vi "phase_shift.vi"(8 "reference":refnum<vi>, 9 "Points in Cycle":i32, 10 "Array 2":dbl[](array[numeric]), 11 "Array 1":dbl[](array[numeric])) -> (3 "Phase Shift":dbl)   [LabVIEW 2020]
doc: "Calculates the phase difference of two input arrays\ninput: two one-dimensional arrays, amount of points within one wave, waveform chart reference\noutput: phase difference"
uses:
  <vilib>/Analysis/5stat.llb/RMS (DBL).vi
  <vilib>/Analysis/NI_AALPro.lvlib
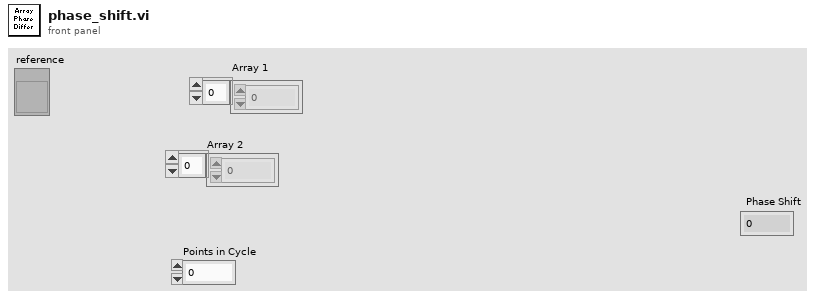
[diagram p1: front panel]
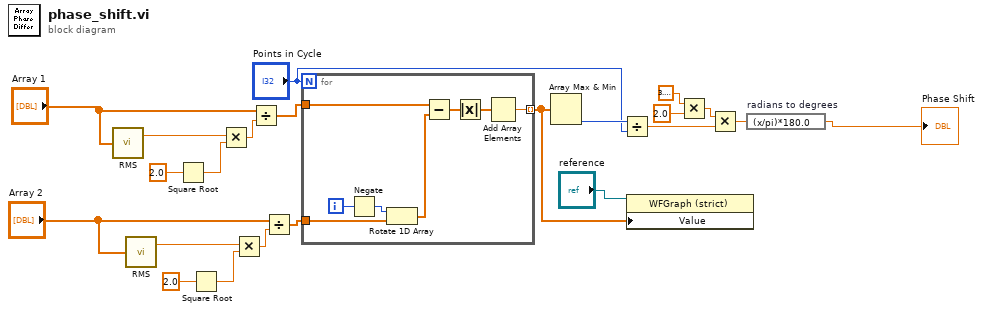
[diagram p0: block diagram]
diagram:
  n1 = call-poly <vilib>:"RMS.vi"("X"="Array 1") -> ("rms value"=w14:dbl)  [unwired: 1 out]
  n2 = call-poly <vilib>:"RMS.vi"("X"="Array 2") -> ("rms value"=w8:dbl)  [unwired: 1 out]
  n3 = Square Root(x=2.0) -> (sqrt(x)=w15:dbl)
  n4 = Square Root(x=2.0) -> (sqrt(x)=w9:dbl)
  n5 = Multiply(x=w14, y=w15) -> (x*y=w12:dbl)
  n6 = Multiply(x=w8, y=w9) -> (x*y=w7:dbl)
  n7 = Divide(x="Array 1", y=w12) -> (x/y=w11:dbl[])
  n8 = Divide(x="Array 2", y=w7) -> (x/y=w5:dbl[])
  n9 = for {
    N: "Points in Cycle" -> [_]
    tunnel: w11 -> [w30]
    tunnel: [w26] -> w2 mode=indexing
    tunnel: w5 -> [w28]
    i -> [w23]
    n10 = Negate(x=w23) -> (-x=w24:i32)
    n11 = Rotate 1D Array(1:w28, 2:w24) -> (0:w25:dbl[])
    n12 = Subtract(x=w30, y=w25) -> (x-y=w29:dbl[])
    n13 = Absolute Value(x=w29) -> (abs(x)=w27:dbl[])
    n14 = Add Array Elements(numeric array=w27) -> (sum=w26:dbl)
  }
  n15 = Array Max & Min(array=w2) -> (min index (indices)=w17:i32)  [unwired: 3 out]
  n16 = Divide(x=w17, y="Points in Cycle") -> (x/y=w18:dbl)
  n17 = property on="Property Node" class="WFGraph (strict)"(reference="reference", "Value"=w2) -> ()  [unwired: 1 in, 2 out]
  n18 = Multiply(x=3.141592653589793, y=2.0) -> (x*y=w21:dbl)
  n19 = Multiply(x=w21, y=w18) -> (x*y=w22:dbl)
  n20 = expression code="(x/pi)*180.0" "radians to degrees"(w22) -> (→"Phase Shift":dbl)
